vi "GlobalVars.vi"() -> ()   [LabVIEW 2016]
panel:
  out "On Target":bool
  out "Turret Fault":bool
  out "Hood Pos":dbl
  out "Wheel Speed":dbl
  out "Intake Chris":bool
  out "Intake Matt":bool
  out "Vision Enabled":bool
  out "Jetson Online":bool
  out "TurretPos":dbl(slide)=2.0140350877192983 scale=-2.0..6.0 scale format="%#_2e"
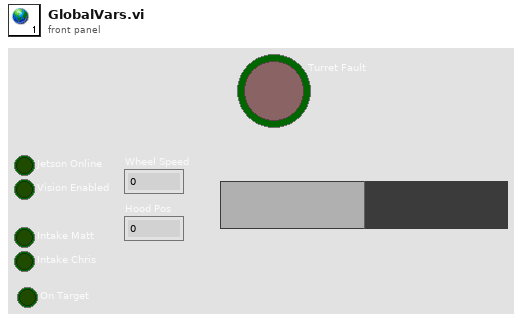
[diagram p1: front panel]
diagram:
